vi "geve-dialog_check_com_port.vi"(10 "Application Message":string, 11 "Runtime Data in":T2={"GEVE Ventilator Monitoring Data"={"On/Off"=FALSE, "Error Ack"=FALSE, "bpm"=0.0, "VT"=0.0, "IE"=0.0, "PEEP"=0.0, "Pressure"=0.0, "Plateau Pressure"=0.0, "Motor Position"=0.0, "Alarm P High"=FALSE, "Alarm P Low"=FALSE, "Alarm Init"=FALSE}, "Serial Port Configuration"={"timeout (ms)"=0, "VISA resource name"="", "baud rate"=0, "max expected byte count"=128}, "Serial Read Return Count"=0, "Read Buffer"="", "Communication Timeout?"=FALSE, "com-refs"={"msg-self Q"=refnum, "gui stop event"=refnum}}) -> (1 "Updated Serial Port Configuration":T1={"timeout (ms)"=0, "VISA resource name"="", "baud rate"=0, "max expected byte count"=128}, 2 "Retry?":bool, 3 "Runtime Data out":T2={"GEVE Ventilator Monitoring Data"={"On/Off"=FALSE, "Error Ack"=FALSE, "bpm"=0.0, "VT"=0.0, "IE"=0.0, "PEEP"=0.0, "Pressure"=0.0, "Plateau Pressure"=0.0, "Motor Position"=0.0, "Alarm P High"=FALSE, "Alarm P Low"=FALSE, "Alarm Init"=FALSE}, "Serial Port Configuration"={"timeout (ms)"=0, "VISA resource name"="", "baud rate"=0, "max expected byte count"=128}, "Serial Read Return Count"=0, "Read Buffer"="", "Communication Timeout?"=FALSE, "com-refs"={"msg-self Q"=refnum, "gui stop event"=refnum}})   [LabVIEW 2018]
doc: "pop up dialog box so the user can changes the com port settings ( com port and baud rate) if those ones generated an error ( wrong config)"
uses:
  geve-runtime_data_cluster.ctl
  geve-monitoring_data_cluster.ctl
  geve-serial_config_cluster.ctl
  geve-com_ref_cluster.ctl
  geve-message_cluster.ctl
panel:
  in  "Baud Rate":u32=9600
  in  "Quit Button":bool
  in  "Retry Button":bool
  in  "COM Port":refnum<visa-resource-name>
  # "Please check if the Arduino is properly connected and check that you're using the correct COM port."
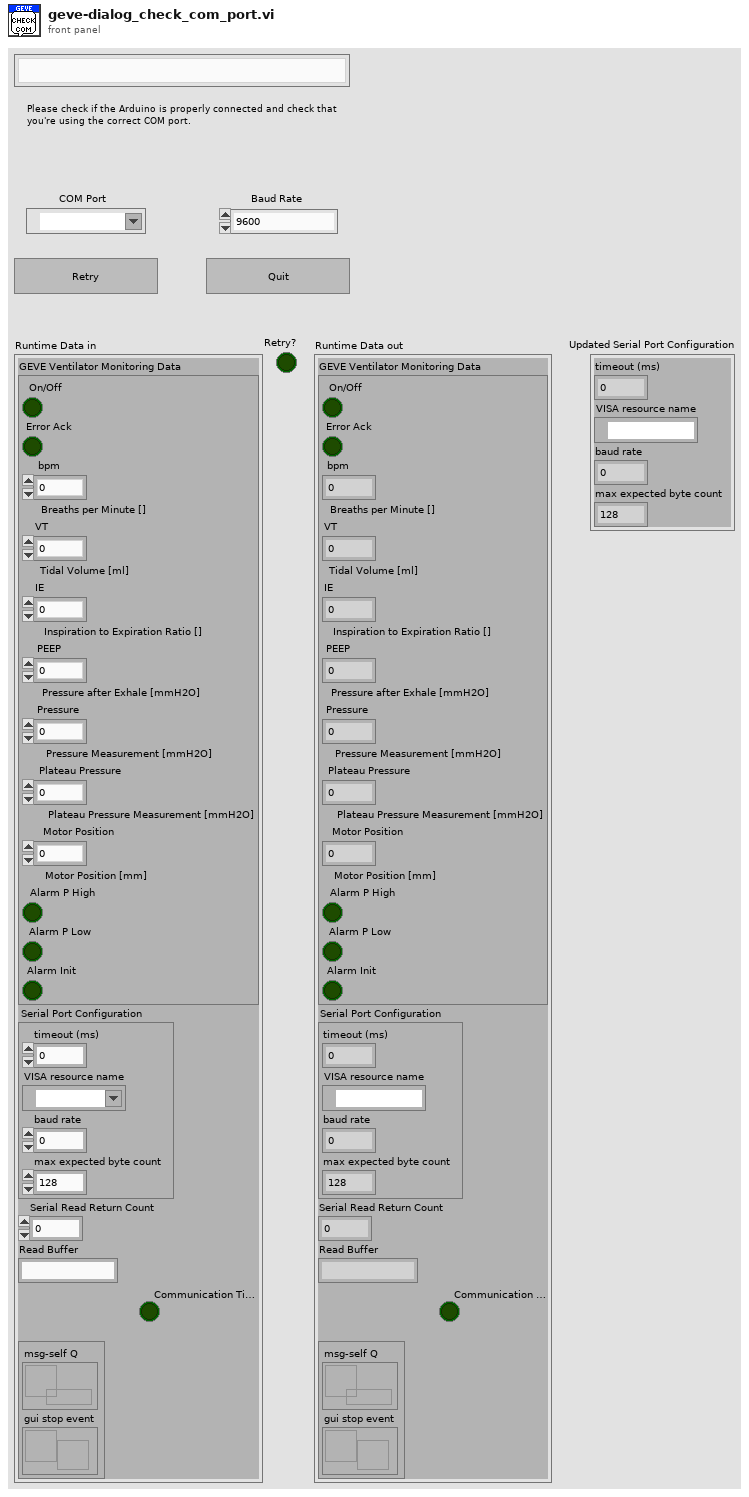
[diagram p1: front panel]
types:
  T1 = typedef "geve-serial_config_cluster.ctl" = cluster{"timeout (ms)":u32, "VISA resource name":refnum<visa-resource-name>, "baud rate":u32, "max expected byte count":u32}
  T2 = typedef "geve-runtime_data_cluster.ctl" = cluster{"GEVE Ventilator Monitoring Data":T3, "Serial Port Configuration":T1, "Serial Read Return Count":u32, "Read Buffer":string, "Communication Timeout?":bool, "com-refs":T4}
  T3 = typedef "geve-monitoring_data_cluster.ctl" = cluster{"On/Off":bool, "Error Ack":bool, "bpm":dbl, "VT":dbl, "IE":dbl, "PEEP":dbl, "Pressure":dbl, "Plateau Pressure":dbl, "Motor Position":dbl, "Alarm P High":bool, "Alarm P Low":bool, "Alarm Init":bool}
  T4 = typedef "geve-com_ref_cluster.ctl" = cluster{"msg-self Q":refnum<queue>, "gui stop event":refnum<user-event>}
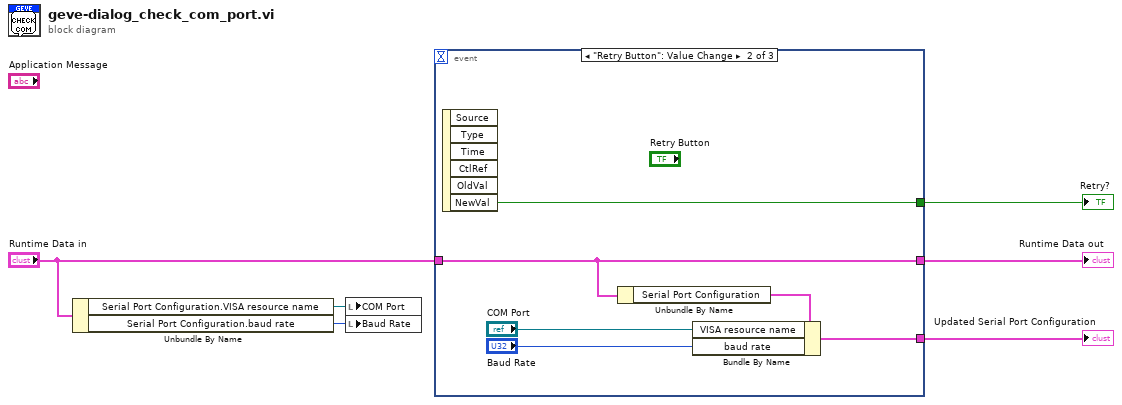
[diagram p0: block diagram]
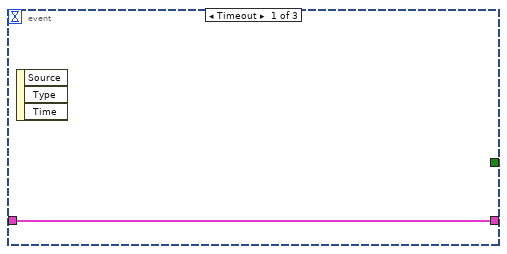
[diagram p2: hidden frame]
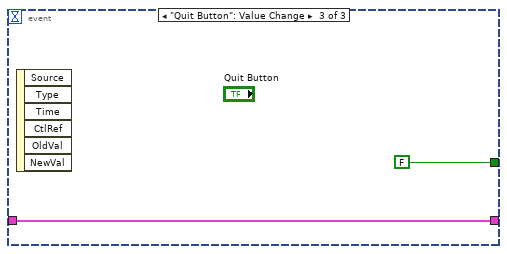
[diagram p3: hidden frame]
diagram:
  n1 = Unbundle By Name("Runtime Data in") -> ("Serial Port Configuration.VISA resource name"=w3:refnum<visa-resource-name>, "Serial Port Configuration.baud rate"=w2:u32)
  n2 = local write "COM Port"(w3) -> ()
  n3 = local write "Baud Rate"(w2) -> ()
  n4 = event shown="[1] \"Retry Button\": Value Change" {
    selector: _ -> [_ _ _]
    dyn-events: _ -> [_ _ _]
    timeout: _ -> [_ _ _]
    tunnel: [_ w13 FALSE ("NewVal")] -> w6
    tunnel: [w7 w10 w14] -> w5
    tunnel: "Runtime Data in" -> [w7 w10 w14]
    tunnel: [_ w8 _] -> w1
    event Timeout {
      n5 = event-data() -> ()  [unwired: 1 in, 3 out]
    }
    event "Retry Button": Value Change {
      n6 = event-data() -> ("NewVal"=w13:bool)  [unwired: 1 in, 5 out]
      n7 = Unbundle By Name(w10) -> ("Serial Port Configuration"=w9:T1)
      n8 = Bundle By Name(cluster=w9, "VISA resource name"="COM Port", "baud rate"="Baud Rate") -> (w8:T1)
    }
    event "Quit Button": Value Change {
      n9 = event-data() -> ()  [unwired: 1 in, 6 out]
    }
  }
  "Retry?" <- w6
  "Runtime Data out" <- w5
  "Updated Serial Port Configuration" <- w1
